vi "DefendAreaTacticVSS.vi"(7 "First call?":bool=TRUE, 8 "error in (no error)":errorcluster, 9 "Game in":refnum<class "Game.lvclass">, 10 "Robot":refnum<class "Robot.lvclass">, 11 "DefendAreaTacticVSS in":refnum<class "DefendAreaTacticVSS.lvclass">) -> (0 "error out":errorcluster, 2 "Robot out":refnum<class "Robot.lvclass">, 3 "DefendAreaTacticVSS out":refnum<class "DefendAreaTacticVSS.lvclass">)   [LabVIEW 2020, in "DefendAreaTacticVSS.lvclass"]
uses:
  DefendAreaTacticVSS.lvclass
  C:/Users/lucio/Desktop/Horie/ROBOIME/VSS_AI/Tactic_class/Tactic.lvclass
  Robot_class/Robot.lvclass
  Game_class/Game.lvclass
  Robot_class/tactics.ctl
  Tactic_class/Tactic.lvclass/Tactic.ctl
  Game_class/Game.lvclass/Game.ctl
  Robot_class/Robot.lvclass/Robot.ctl
  Skillbook_class/Skillbook.lvclass/Skillbook.ctl
  Game_class/Read BallRef.vi
  Game_class/Read FieldRef.vi
  Robot_class/Read dest_x.vi
  Robot_class/Read dest_y.vi
  Robot_class/Write dest_x.vi
  Robot_class/Write dest_y.vi
  Skillbook_class/Read HaltSkill.vi
  Tactic_class/Read Skillbook.vi
  Robot_class/Write tactic.vi
  Skillbook_class/Skillbook.lvclass
  KickSkillVSS_class/KickSkillVSS.lvclass
  PenaltyPosSkillVSS_class/PenaltyPosSkillVSS.lvclass
  BallDispPosSkillVSS_class/BallDispPosSkillVSS.lvclass
  BallToGoalSkillVSS_class/BallToGoalSkillVSS.lvclass
  GoToBallSkillVSS_class/GoToBallSkillVSS.lvclass
  DefBallPosSkillVSS_class/DefBallPosSkillVSS.lvclass
  HaltSkill_class/HaltSkill.lvclass
  KeeperDefPosSkillVSS_class/KeeperDefPosSkillVSS.lvclass
  GoToBallKeeperSkillVSS_class/GoToBallKeeperSkillVSS.lvclass
  RotateWallSkillVSS_class/RotateWallSkillVSS.lvclass
  Ball_class/Ball.lvclass
  Field_class/Field.lvclass
panel:
  out "x .or. y?":bool
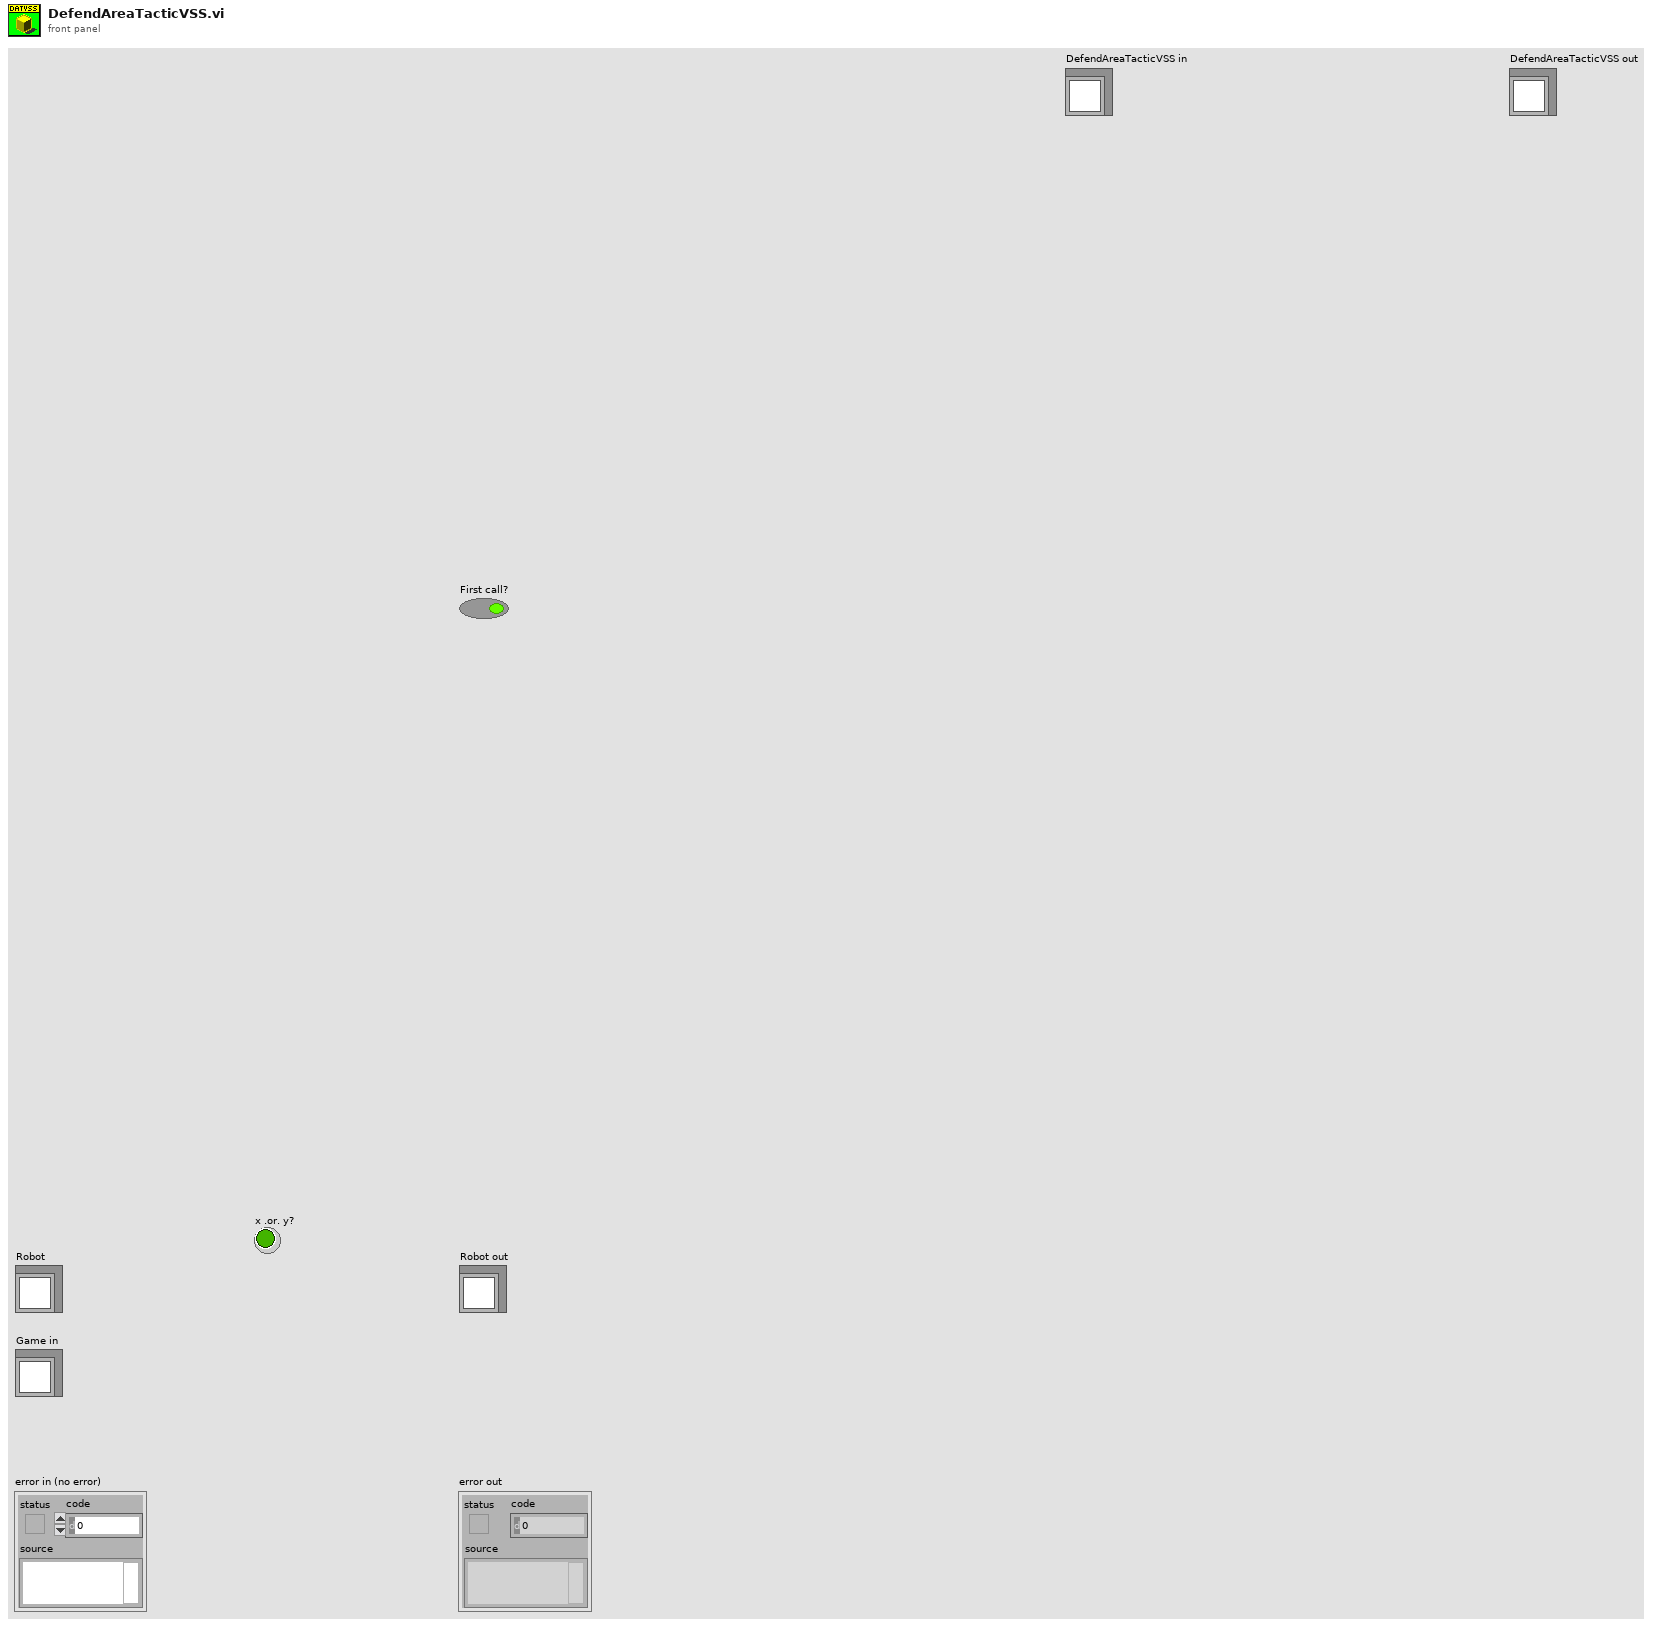
[diagram p1: front panel]
types:
  T1 = enum16{"Exit", "Kick", "DefBallPos", "GoToBall", "Halt"}
  T2 = typedef "tactics.ctl" = enum16{"ReceivePassInFuturePoint", "Roller", "PrepareRollToPassRollerGoTo", "PrepareRollToPassReceiverGoTo", "WaitRoll", "PositionToRoll", "PenaltyAttacker", "PassObserver", "PenaltyDefense", "TableReceiverTactic", "Test", "DefendGoal", "Marker", "FollowAttacker", "DefendArea", "Shoot", "AttackerAimGoal", "AttackerBallOutOfField", "AttackerBlock", "AttackerStop", "Duelist", "Halt", "ZigZag", "GoTo", "Timeout", "KickToPassReceiver", "PositionToReceivePass", "DefendAreaVSS", "DefendGoalVSS", "KickVSS", "AttackVSS", "DispBallVSS", "PenaltyAttackVSS", "WaitPass"}
  T3 = cluster{"KickSkillVSS":refnum<class "KickSkillVSS.lvclass">, "PenaltyPosSkillVSS":refnum<class "PenaltyPosSkillVSS.lvclass">, "BallDispPosSkillVSS":refnum<class "BallDispPosSkillVSS.lvclass">, "BallToGoalSkillVSS":refnum<class "BallToGoalSkillVSS.lvclass">, "GoToBallSkillVSS":refnum<class "GoToBallSkillVSS.lvclass">, "DefBallPosSkillVSS":refnum<class "DefBallPosSkillVSS.lvclass">, "HaltSkill":refnum<class "HaltSkill.lvclass">, "KeeperDefPosSkillVSS":refnum<class "KeeperDefPosSkillVSS.lvclass">, "GoToBallKeeperSkillVSS":refnum<class "GoToBallKeeperSkillVSS.lvclass">, "RotateWallSkillVSS":refnum<class "RotateWallSkillVSS.lvclass">}
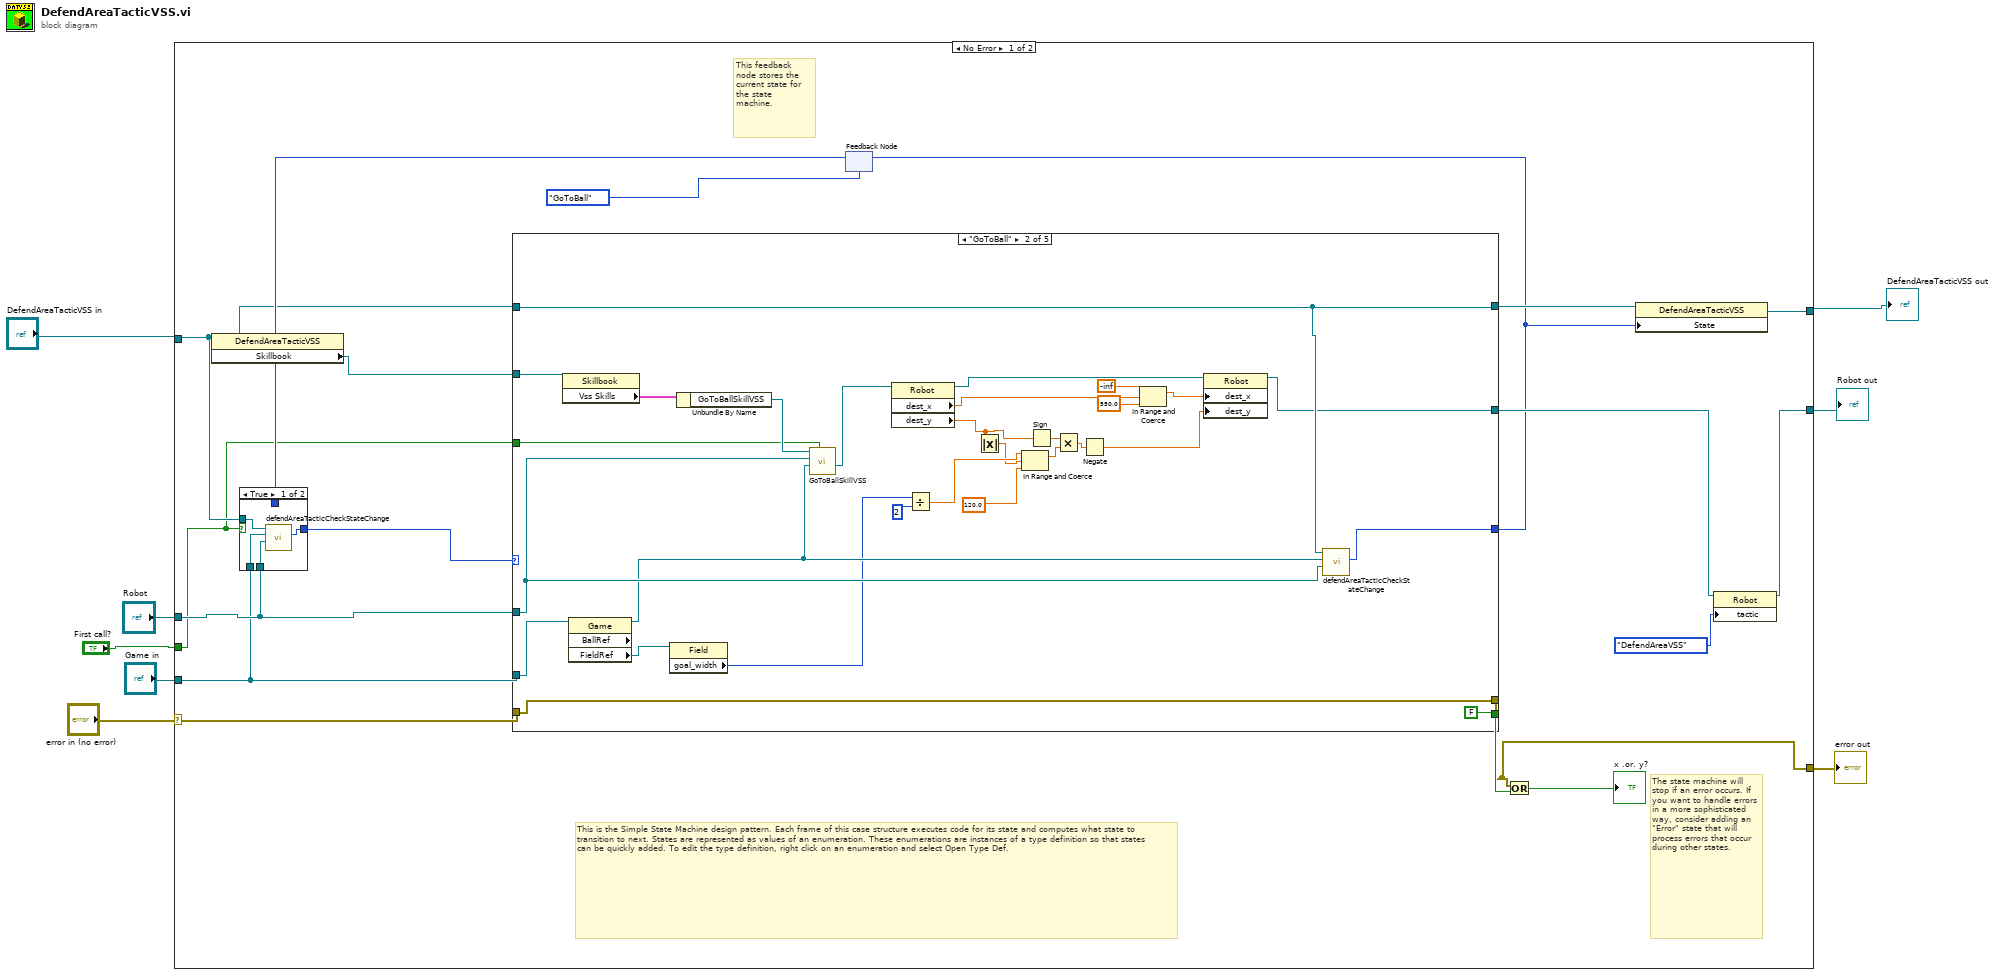
[diagram p0: block diagram]
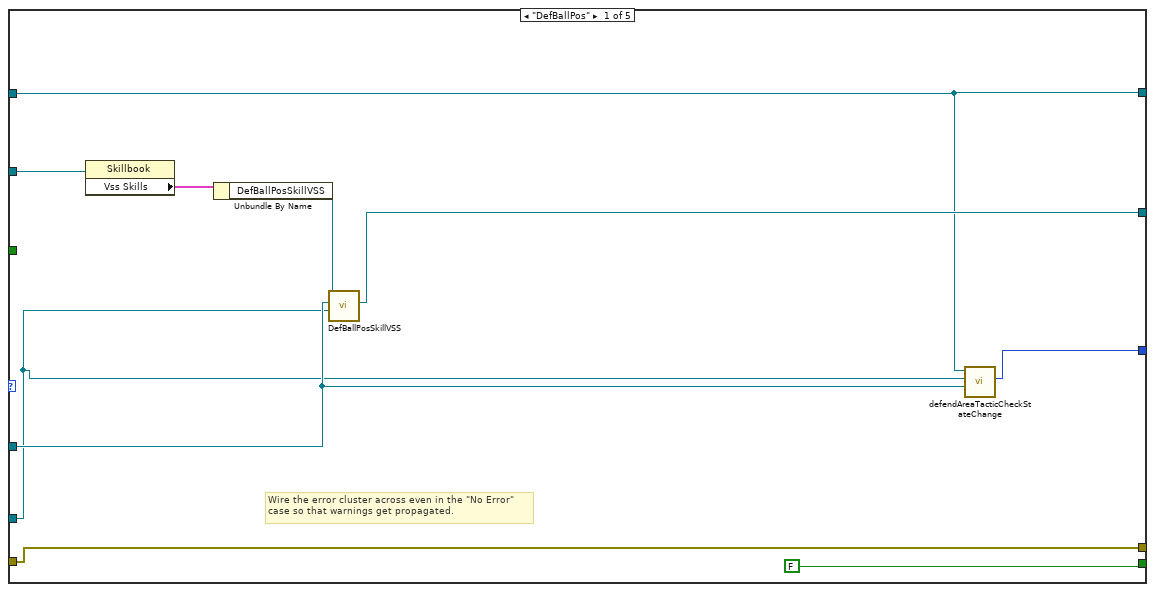
[diagram p2: hidden frame]
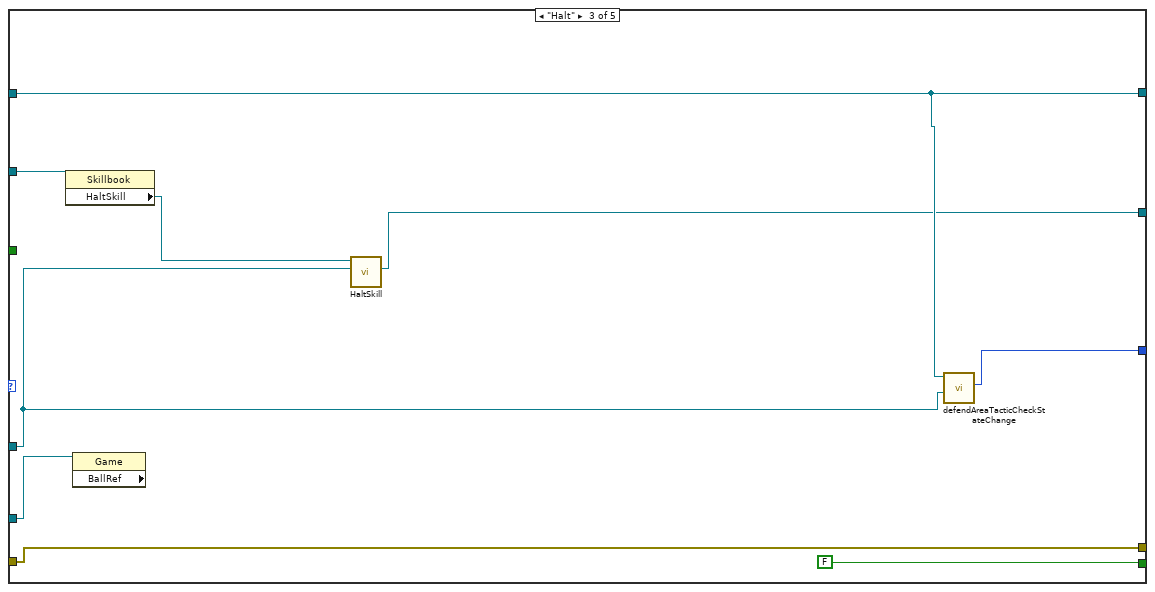
[diagram p3: hidden frame]
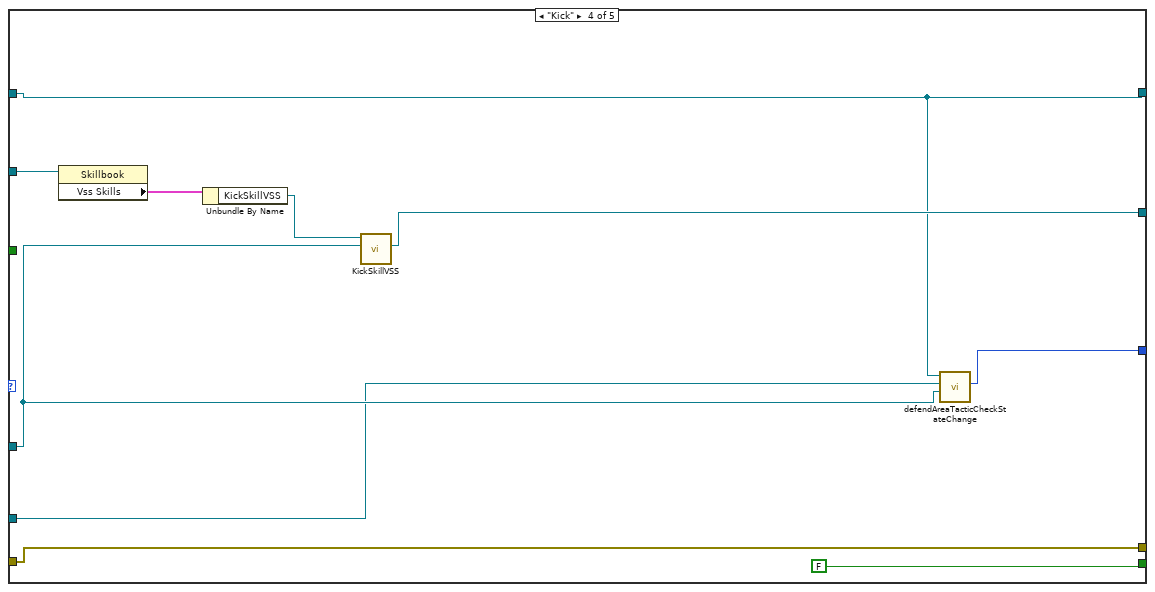
[diagram p4: hidden frame]
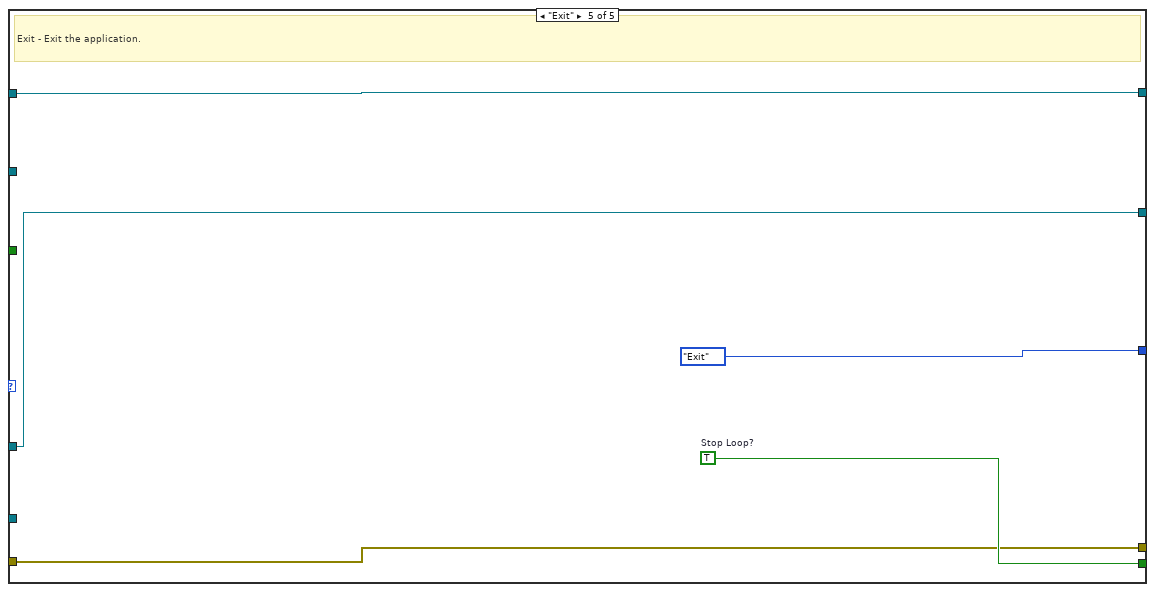
[diagram p5: hidden frame]
diagram:
  n1 = case shown="No Error" "error in (no error)" {
    selector: "error in (no error)" -> [w22 w97]
    tunnel: [w21 w97] -> w7
    tunnel: [w20 w96] -> w1
    tunnel: "DefendAreaTacticVSS in" -> [w14 w96]
    tunnel: "Robot" -> [w13 w95]
    tunnel: "Game in" -> [w12 _]
    tunnel: [w17 w95] -> w4
    tunnel: "First call?" -> [w9 _]
    frame No Error {
      # "The state machine will stop if an error occurs. If you want to handle errors in a more sophisticated way, consider adding an \"Error\" state that will process errors that occur during other states."
      # "This feedback node stores the current state for the state machine."
      # "This is the Simple State Machine design pattern. Each frame of this case structure executes code for its state and computes what state to transition to next. States are represented as values of an enumeration. These enumerations are instances of a type definition so that states can be quickly added. To edit the type definition, right click on an enumeration and select Open Type Def."
      n2 = property class="DefendAreaTacticVSS"(reference=w14) -> ("Skillbook"=w24:refnum<class "Skillbook.lvclass">)  [unwired: 1 in, 2 out]
      n3 = feedback #1(T1."GoToBall" ("State")) -> (w16:T1)
      n4 = case shown="True" w9 {
        tunnel: [w92 w94] -> w15
        tunnel: w16 -> [_ w94]
        tunnel: w14 -> [w93 _]
        tunnel: w13 -> [w91 _]
        tunnel: w12 -> [w90 _]
        frame True {
          n5 = call "defendAreaTacticCheckStateChange.vi"("Robot In"=w91, "Game in"=w90, "DefendAreaTacticVSS in"=w93) -> ("State"=w92:T1)  [unwired: 6 in, 2 out]
        }
        frame False {
        }
      }
      n6 = case shown="\"GoToBall\"" w15 {
        tunnel: [FALSE FALSE FALSE FALSE w89] -> w26
        tunnel: w24 -> [w35 w64 w74 w83 _]
        tunnel: w13 -> [w29 w59 w68 w77 w88]
        tunnel: [w32 w52 w69 w79 w88] -> w18
        tunnel: [w31 w61 w71 w78 w87] -> w23
        tunnel: w14 -> [w31 w61 w71 w78 w87]
        tunnel: w12 -> [w28 w60 w70 w76 _]
        tunnel: [w34 w63 w73 w81 w86] -> w21
        tunnel: w22 -> [w34 w63 w73 w81 w86]
        tunnel: [w27 w57 w67 w75 T1."Exit" ("State")] -> w10
        tunnel: w9 -> [_ w55 _ _ _]
        frame "DefBallPos" {
          # "Wire the error cluster across even in the \"No Error\"\ncase so that warnings get propagated."
          n7 = property class="Skillbook"(reference=w35) -> ("Vss Skills"=w36:T3)  [unwired: 1 in, 2 out]
          n8 = Unbundle By Name(w36) -> ("DefBallPosSkillVSS"=w30:refnum<class "DefBallPosSkillVSS.lvclass">)
          n9 = call-dynamic "DefBallPosSkillVSS.vi"("Game"=w28, "Robot in"=w29, "DefBallPosSkillVSS in"=w30) -> ("Robot out"=w32:refnum<class "Robot.lvclass">)  [unwired: 6 in, 2 out]
          n10 = call "defendAreaTacticCheckStateChange.vi"("Robot In"=w29, "Game in"=w28, "DefendAreaTacticVSS in"=w31) -> ("State"=w27:T1)  [unwired: 6 in, 2 out]
        }
        frame "GoToBall" {
          n11 = property class="Skillbook"(reference=w64) -> ("Vss Skills"=w65:T3)  [unwired: 1 in, 2 out]
          n12 = property class="Game" props=["BallRef", "FieldRef"](reference=w60) -> (reference out=w58:refnum<class "Game.lvclass">, "FieldRef"=w51:refnum<class "Field.lvclass">)  [unwired: 1 in, 2 out]
          n13 = property class="Field"(reference=w51) -> ("goal_width"=w50:i32)  [unwired: 1 in, 2 out]
          n14 = Unbundle By Name(w65) -> ("GoToBallSkillVSS"=w56:refnum<class "GoToBallSkillVSS.lvclass">)
          n15 = call "GoToBallSkillVSS.vi"("First call?"=w55, "Game"=w58, "Robot in"=w59, "GoToBallSkillVSS in"=w56) -> ("Robot out"=w54:refnum<class "Robot.lvclass">)  [unwired: 5 in, 2 out]
          n16 = property class="Robot"(reference=w54) -> (reference out=w53:refnum<class "Robot.lvclass">, "dest_x"=w39:dbl, "dest_y"=w46:dbl)  [unwired: 1 in, 1 out]
          n17 = Divide(x=w50, y=2) -> (x/y=w48:dbl)
          n18 = Absolute Value(x=w46) -> (abs(x)=w47:dbl)
          n19 = In Range and Coerce(upper limit=w48, x=w47, lower limit=120.0) -> (coerced(x)=w44:dbl)  [unwired: 1 out]
          n20 = Sign(1:w46) -> (0:w45:dbl)
          n21 = Multiply(x=w45, y=w44) -> (x*y=w42:dbl)
          n22 = Negate(x=w42) -> (-x=w41:dbl)
          n23 = In Range and Coerce(upper limit=-inf, x=w39, lower limit=550.0) -> (coerced(x)=w40:dbl)  [unwired: 1 out]
          n24 = property class="Robot"(reference=w53, "dest_x"=w40, "dest_y"=w41) -> (reference out=w52:refnum<class "Robot.lvclass">)  [unwired: 1 in, 1 out]
          n25 = call "defendAreaTacticCheckStateChange.vi"("Robot In"=w59, "Game in"=w58, "DefendAreaTacticVSS in"=w61) -> ("State"=w57:T1)  [unwired: 6 in, 2 out]
        }
        frame "Halt" {
          n26 = property class="Skillbook"(reference=w74) -> ("HaltSkill"=w66:refnum<class "HaltSkill.lvclass">)  [unwired: 1 in, 2 out]
          n27 = property class="Game" props=["BallRef"](reference=w70) -> ()  [unwired: 1 in, 3 out]
          n28 = call-dynamic "HaltSkill.vi"("Robot"=w68, "HaltSkill in"=w66) -> ("Robot out"=w69:refnum<class "Robot.lvclass">)  [unwired: 7 in, 2 out]
          n29 = call "defendAreaTacticCheckStateChange.vi"("Robot In"=w68, "DefendAreaTacticVSS in"=w71) -> ("State"=w67:T1)  [unwired: 7 in, 2 out]
        }
        frame "Kick" {
          n30 = property class="Skillbook"(reference=w83) -> ("Vss Skills"=w84:T3)  [unwired: 1 in, 2 out]
          n31 = Unbundle By Name(w84) -> ("KickSkillVSS"=w80:refnum<class "KickSkillVSS.lvclass">)
          n32 = call-dynamic "KickSkillVSS.vi"("Robot"=w77, "KickSkillVSS in"=w80) -> ("Robot out"=w79:refnum<class "Robot.lvclass">)  [unwired: 7 in, 2 out]
          n33 = call "defendAreaTacticCheckStateChange.vi"("Robot In"=w77, "Game in"=w76, "DefendAreaTacticVSS in"=w78) -> ("State"=w75:T1)  [unwired: 6 in, 2 out]
        }
        frame "Exit" {
          w89 = TRUE  # Stop Loop?
          # "Exit - Exit the application."
        }
      }
      n34 = feedback-in #1(w10) -> ()
      n35 = Or(x=w21, y=w26) -> (x .or. y?=→"x .or. y?":bool)
      n36 = property class="DefendAreaTacticVSS"(reference=w23, "State"=w10) -> (reference out=w20:refnum<class "DefendAreaTacticVSS.lvclass">)  [unwired: 1 in, 1 out]
      n37 = property class="Robot"(reference=w18, "tactic"=tactics."DefendAreaVSS") -> (reference out=w17:refnum<class "Robot.lvclass">)  [unwired: 1 in, 1 out]
    }
    frame Error {
    }
  }
  "DefendAreaTacticVSS out" <- w1
  "error out" <- w7
  "Robot out" <- w4
